vi "2ballzauto.vi"() -> ()   [LabVIEW 2013]
uses:
  drive/drive_inputs.ctl
  flinger/flinger_inputs.ctl
  roller/roller_inputs.ctl
  catch/catch_inputs.ctl
  inputs.ctl
panel:
  in  "Inputs":T1
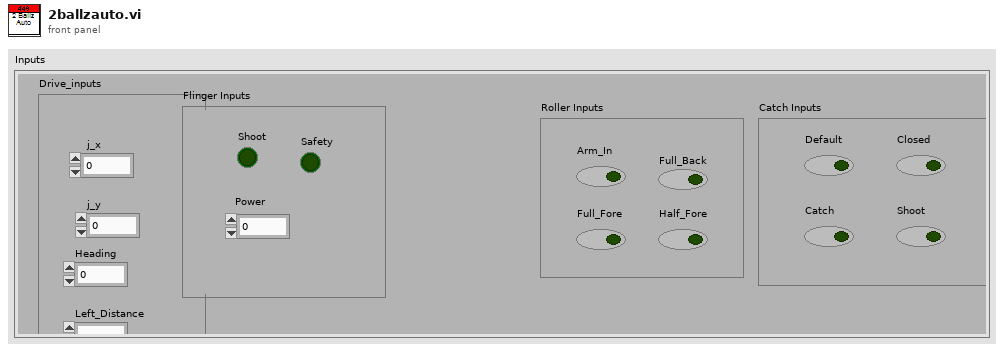
[diagram p1: front panel]
types:
  T1 = typedef "inputs.ctl" = cluster{"Drive_inputs":T2, "Flinger Inputs":T3, "Roller Inputs":T4, "Catch Inputs":T5}
  T2 = typedef "drive_inputs.ctl" = cluster{"j_x":dbl, "j_y":dbl, "Heading":dbl, "Left_Distance":dbl, " Right_Distance":dbl}
  T3 = typedef "flinger_inputs.ctl" = cluster{"Shoot":bool, "Power":dbl, "Safety":bool}
  T4 = typedef "roller_inputs.ctl" = cluster{"Arm_In":bool, "Full_Fore":bool, "Full_Back":bool, "Half_Fore":bool}
  T5 = typedef "catch_inputs.ctl" = cluster{"Default":bool, "Closed":bool, "Catch":bool, "Shoot":bool}
  T6 = typedef "WPI_EncoderDevRef.ctl" = cluster{"DevStatus":errorcluster, "EncoderIndex":T7, "CounterIndex":T8, "DistancePerCount":dbl, "Decoding Type":T9}
  T7 = typedef "FPGA_EncoderIdx.ctl" = enum8{"Enc 0", "Enc 1", "Enc 2", "Enc 3", "Invalid"}
  T8 = typedef "FPGA_CounterCtrSystemIndex.ctl" = enum8{"Ctr 0", "Ctr 1", "Ctr 2", "Ctr 3", "Ctr 4", "Ctr 5", "Ctr 6", "Ctr 7", "Invalid"}
  T9 = typedef "WPI_EncoderType.ctl" = enum16{"1x", "2x", "4x"}
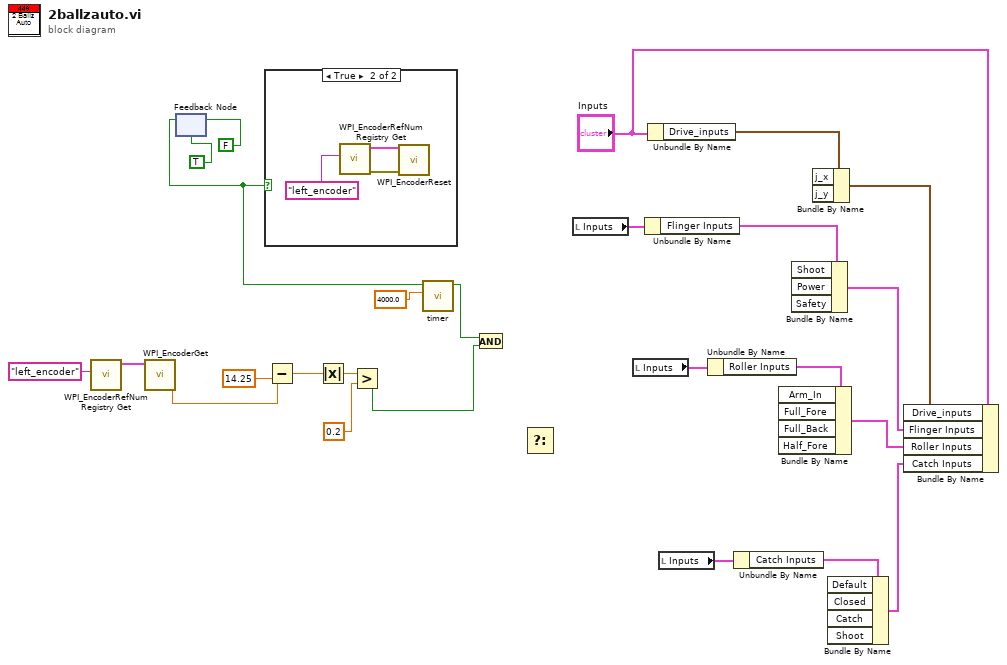
[diagram p0: block diagram]
diagram:
  n1 = call <vilib>:"WPI_EncoderRefNum Registry Get.vi"("refnum name"="left_encoder") -> ("EncoderDevRef"=w22:T6)  [unwired: 9 in, 1 out]
  n2 = call <vilib>:"WPI_EncoderGet.vi"("EncoderDevRef"=w22) -> ("Distance"=w19:dbl)  [unwired: 5 in, 5 out]
  n3 = feedback-in #1(FALSE) -> ()
  n4 = feedback #1(TRUE) -> (w21:bool)
  n5 = case shown="True" w21 {
    frame False {
    }
    frame True {
      n6 = call <vilib>:"WPI_EncoderRefNum Registry Get.vi"("refnum name"="left_encoder") -> ("error out"=w27:errorcluster, "EncoderDevRef"=w28:T6)  [unwired: 9 in]
      n7 = call <vilib>:"WPI_EncoderReset.vi"("error in (no error)"=w27, "EncoderDevRef"=w28) -> ()  [unwired: 8 in, 2 out]
    }
  }
  n8 = Subtract(x=w19, y=14.25) -> (x-y=w17:dbl)
  n9 = Absolute Value(x=w17) -> (abs(x)=w16:dbl)
  n10 = Greater?(x=w16, y=0.2) -> (0:w13:bool)
  n11 = call "timer.vi"("Time"=4000.0, "Set"=w21) -> ("Out"=w14:bool)  [unwired: 9 in]
  n12 = And(x=w14, y=w13) -> ()  [unwired: 1 out]
  n13 = Select() -> ()  [unwired: 3 in, 1 out]
  n14 = local read "Inputs"() -> (w9:T1)
  n15 = local read "Inputs"() -> (w6:T1)
  n16 = Unbundle By Name(w9) -> ("Flinger Inputs"=w8:T3)
  n17 = Unbundle By Name("Inputs") -> ("Drive_inputs"=w12:T2)
  n18 = local read "Inputs"() -> (w3:T1)
  n19 = Unbundle By Name(w6) -> ("Roller Inputs"=w5:T4)
  n20 = Unbundle By Name(w3) -> ("Catch Inputs"=w2:T5)
  n21 = Bundle By Name(cluster=w5) -> (w4:T4)  [unwired: 4 in]
  n22 = Bundle By Name(cluster=w8) -> (w7:T3)  [unwired: 3 in]
  n23 = Bundle By Name(cluster=w12) -> (w11:T2)  [unwired: 2 in]
  n24 = Bundle By Name(cluster=w2) -> (w1:T5)  [unwired: 4 in]
  n25 = Bundle By Name(cluster="Inputs", "Drive_inputs"=w11, "Flinger Inputs"=w7, "Roller Inputs"=w4, "Catch Inputs"=w1) -> ()  [unwired: 1 out]
